vi "Write Time Stamp of Next.vi"(8 "error in (no error)":errorcluster, 10 "Time Stamp of Next":timestamp, 11 "ARecurrence in":refnum<class "ARecurrence.lvclass">) -> (0 "error out":errorcluster, 3 "ARecurrence out":refnum<class "ARecurrence.lvclass">)   [LabVIEW 2020, in "ARecurrence.lvclass"]
uses:
  ARecurrence.lvclass
  ARecurrence.lvclass/ARecurrence.ctl
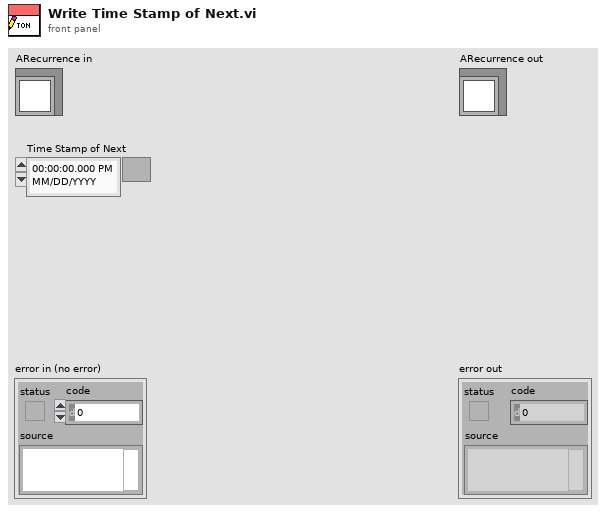
[diagram p1: front panel]
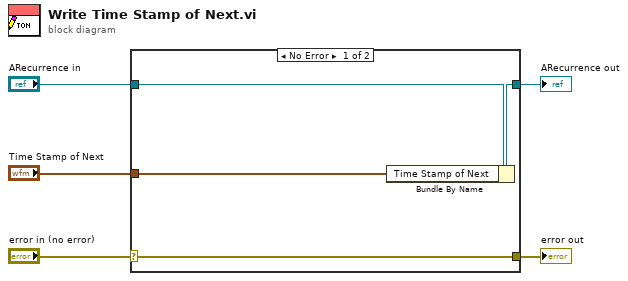
[diagram p0: block diagram]
diagram:
  n1 = case shown="No Error" "error in (no error)" {
    selector: "error in (no error)" -> [w9 w10]
    tunnel: [w9 w10] -> w4
    tunnel: [w7 w11] -> w2
    tunnel: "ARecurrence in" -> [w8 w11]
    tunnel: "Time Stamp of Next" -> [w6 _]
    frame No Error {
      n2 = Bundle By Name(cluster=w8, "Time Stamp of Next"=w6) -> (w7:refnum<class "ARecurrence.lvclass">)
    }
    frame Error {
    }
  }
  "error out" <- w4
  "ARecurrence out" <- w2
